vi "Unicode Path With LabVIEW File IO Example.vi"() -> ()   [LabVIEW 2020]
doc: "This example demonstrates creating and writing unicode paths using LabVIEW's TDMS primitives. This technique can be extended to any LabVIEW file I/O primitives such as config files, xml files, and so on."
uses:
  Unicode/Controls/String Encoding.ctl
  Types/UTF-8 String/UTF-8 String.lvclass/UTF-8 String.ctl
  Types/UTF-8 Path/UTF-8 Path.lvclass/UTF-8 Path.ctl
  adeaac51-e73f-479d-a693-bb7f399b7a58.vi
  c1cbc64f-dc2e-462b-b757-29338a356fe5.vi
  a3fedd63-8064-49e9-9d91-1abce6ab3d35.vi
  fc41487d-943f-4c2f-8ebb-b047207c64a4.vi
  Dialog & User Interface/Polymorphic VIs/Write Control Text/Write 1D String Array Value (UTF-8 String).vi
  3e39073b-8a5d-4733-9d90-f00b4091e0ed.vi
  Unicode/Encode String.vi
  adeaac51-e73f-479d-a693-bb7f399b7a58.vi/b0de225b-b813-4a3f-91fa-b2c78c384815.vi
  adeaac51-e73f-479d-a693-bb7f399b7a58.vi/b1dd94da-e188-4359-85d0-d6693b26af46.vi
  adeaac51-e73f-479d-a693-bb7f399b7a58.vi/2799960a-efad-449d-b375-cc5363f1c370.vi
  adeaac51-e73f-479d-a693-bb7f399b7a58.vi/2ed7adf8-1da0-426c-b32d-a1b4538e7e16.vi
  Types/UTF-8 String/Write Encoded UTF-8 String.vi
  Private/Conversion/Text as Encoded Path.vi
  Private/Conversion/Polymorphic VIs/Text as Encoded Path (UTF-8 String).vi
  Types/UTF-8 Path/Write Encoded UTF-8 Path.vi
  Private/Conversion/Path as Encoded Path.vi
  Private/Conversion/Polymorphic VIs/Path as Encoded Path (LabVIEW Path).vi
  Private/Conversion/Text as Encoded String.vi
  Private/Conversion/Polymorphic VIs/Text as Encoded String (UTF-8 Path).vi
  Private/Conversion/Path as UTF-8 Path.vi
  Private/Conversion/Polymorphic VIs/Path as UTF-8 Path (UTF-8 Path).vi
  Private/Library/gu_create_file.vi
  Private/Library/gu_long_path.vi
  Private/Conversion/Polymorphic VIs/Path as UTF-8 Path (LabVIEW Path).vi
  fc41487d-943f-4c2f-8ebb-b047207c64a4.vi/5269e09c-4216-478e-8686-9fb7d38e224a.vi
  fc41487d-943f-4c2f-8ebb-b047207c64a4.vi/d1f4a45d-6f02-44dd-a40b-2b28d80e6519.vi
  Private/Conversion/String as Encoded String.vi
  Private/Conversion/Polymorphic VIs/String as Encoded String (UTF-8 String).vi
  Private/Library/gu_list_folder.vi
  fc41487d-943f-4c2f-8ebb-b047207c64a4.vi/8eb4f0ed-0012-4550-978e-be3f7301df70.vi
  fc41487d-943f-4c2f-8ebb-b047207c64a4.vi/f7e6584c-01ed-423f-9bcd-660954191d0d.vi
  Private/Conversion/Polymorphic VIs/String as Encoded String (LabVIEW String).vi
  Dialog & User Interface/Polymorphic VIs/Write Control Text/Write 1D String Array Value (UTF-8 String).vi/5206cb6b-04fb-41f5-a37e-29c14f142303.vi
  3e39073b-8a5d-4733-9d90-f00b4091e0ed.vi/cd814f09-858d-41ec-a1ea-d598fdb95b0d.vi
  3e39073b-8a5d-4733-9d90-f00b4091e0ed.vi/cdde7a24-321d-4ebe-8fa8-ef041a4f6d83.vi
  Types/UTF-8 Path/New UTF-8 Path.vi
  Private/Library/gu_delete.vi
  3e39073b-8a5d-4733-9d90-f00b4091e0ed.vi/80924ba4-6f01-46cb-bebd-728ad922c70d.vi
  Private/Conversion/String as UTF-8 String.vi
  Private/Conversion/Polymorphic VIs/String as UTF-8 String (UTF-8 String).vi
  Private/Conversion/Text to UTF-8.vi
  Private/Conversion/Polymorphic VIs/Text to UTF-8 (LabVIEW String).vi
  Private/Conversion/Encoded UTF-8 String to Encoded UTF-16LE String.vi
  Private/Conversion/UTF-8 to Text.vi
  Private/Conversion/Polymorphic VIs/UTF-8 to Text (LabVIEW String).vi
  Private/Conversion/Encoded UTF-16LE String to Encoded UTF-8 String.vi
  Unicode/Prepend BOM.vi
  Types/UTF-8 String/Read Encoded UTF-8 String.vi
  Private/Conversion/Polymorphic VIs/Text to UTF-8 (LabVIEW Path).vi
  Types/UTF-8 Path/Read Encoded UTF-8 Path.vi
  Private/Library/Result To Error.vi
  Private/Memory/Copy String.vi
  fc41487d-943f-4c2f-8ebb-b047207c64a4.vi/5269e09c-4216-478e-8686-9fb7d38e224a.vi/c24c063b-f849-48a1-b323-238a063d7118.vi
  fc41487d-943f-4c2f-8ebb-b047207c64a4.vi/5269e09c-4216-478e-8686-9fb7d38e224a.vi/a2fd6c11-d594-45c9-8624-1f0a1df69df3.vi
  fc41487d-943f-4c2f-8ebb-b047207c64a4.vi/5269e09c-4216-478e-8686-9fb7d38e224a.vi/1fd3173e-d32e-42cb-8f0d-819132eb8e27.vi
  fc41487d-943f-4c2f-8ebb-b047207c64a4.vi/5269e09c-4216-478e-8686-9fb7d38e224a.vi/bb7c39fc-ad8e-447d-bc50-468674bfb562.vi
  fc41487d-943f-4c2f-8ebb-b047207c64a4.vi/8eb4f0ed-0012-4550-978e-be3f7301df70.vi/3a31b270-3bb6-4c58-a256-c5fcc2c98f09.vi
  fc41487d-943f-4c2f-8ebb-b047207c64a4.vi/8eb4f0ed-0012-4550-978e-be3f7301df70.vi/0ec5df2d-ef9b-4f84-a6a8-ffcedd45c4dc.vi
  Private/Conversion/Text as String.vi
  Private/Conversion/Polymorphic VIs/Text as String (UTF-8 Path).vi
  Private/Conversion/Polymorphic VIs/Text as Encoded String (UTF-8 String).vi
  3e39073b-8a5d-4733-9d90-f00b4091e0ed.vi/cd814f09-858d-41ec-a1ea-d598fdb95b0d.vi/9afeabe8-8abe-4536-bea1-05e5a3549c28.vi
  Private/Library/gu_open_file_dialog.vi
  Private/Library/gu_select_folder_dialog.vi
  Private/Conversion/Polymorphic VIs/Text as String (UTF-8 String).vi
  Unicode/SubVIs/Byte Order Marks.vi
  Unicode/Detect BOM.vi
  Private/Memory/Copy String.vi/4d47babd-4a2d-4eb7-b91b-7e707d692665.vi
  Private/Library/gu_free.vi
  Private/Conversion/Polymorphic VIs/Path as Encoded Path (UTF-8 Path).vi
  Private/Library/gu_string_subset.vi
  Private/Library/gu_to_lower_case.vi
  Private/Library/gu_search_split_string.vi
  Private/Conversion/Polymorphic VIs/Text as Encoded String (LabVIEW String).vi
  Unicode/Detect String Encoding.vi
  <vilib>/Utility/error.llb/Error Cluster From Error Code.vi
  Private/Memory/Copy String Array.vi
  Private/User Interface/Write String Array (1D).vi
  Types/UTF-8 String/UTF-8 String.lvclass
  Types/UTF-8 Path/UTF-8 Path.lvclass
  G-Unicode.lvlib
panel:
  out "error out":errorcluster
  out "TDMS Files":string[](array[string])
  # "Instructions:\n1. Run the VI.\n2. Check the TDMS Files contains a list of files with unicode characters."
  # "This example demonstrates creating and writing unicode paths using LabVIEW's TDMS primitives. This technique can be extended to any LabVIEW file I/O primitives such as config files, xml files, and so on.\n\nTo use unicode paths, it must first be converted to an 8.3 short path, which are compatible with any of LabVIEW's file I/O functions.\n\nIn order to convert the unicode path to the 8.3 short path, the file must first exist on disk. This can be achieved using Create File.vim, which accepts unicode paths.\n\nAfter file I/O is complete and the file closed, the short path can be converted back to the long (unicode) path."
  # "G"
  # "-Unicode"
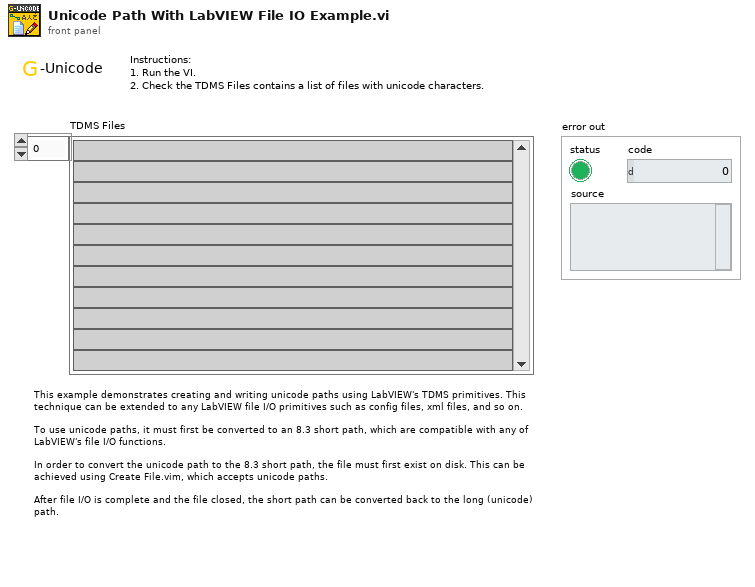
[diagram p1: front panel]
types:
  T1 = typedef "G-Unicode.lvlib/String Encoding.ctl" = enum16{"ANSI", "UTF-8", "UTF-16LE", "UTF-16BE", "Unknown"}
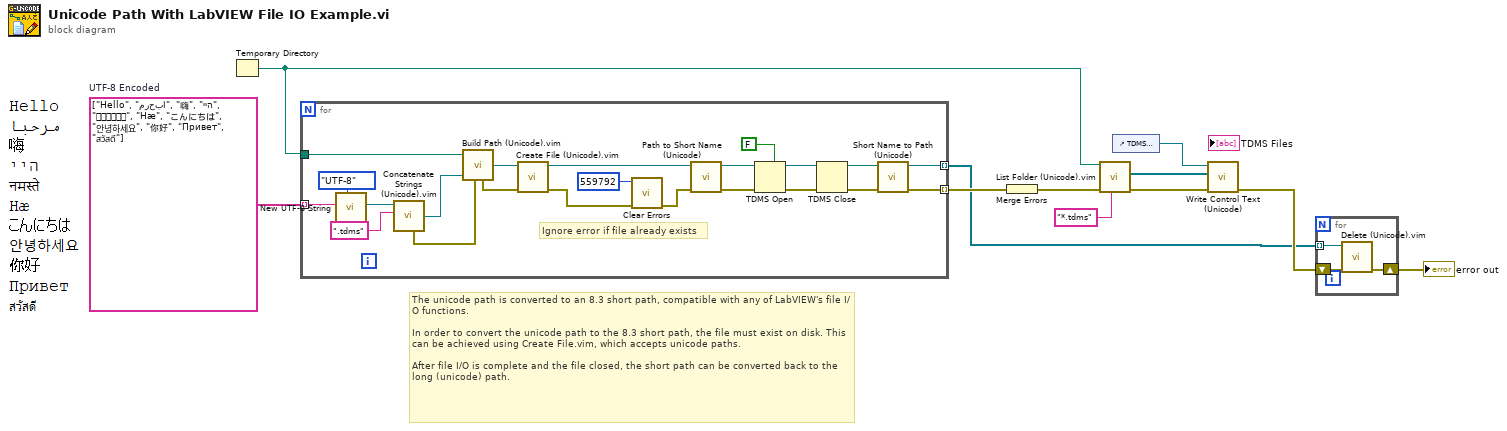
[diagram p0: block diagram]
diagram:
  w6 = string[] ["Hello", "مرحبا", "嗨", "היי", "नमस्ते", "Hæ", "こんにちは", "안녕하세요", "你好", "Привет", "สวัสดี"]  # UTF-8 Encoded
  # "The unicode path is converted to an 8.3 short path, compatible with any of LabVIEW's file I/O functions.\n\nIn order to convert the unicode path to the 8.3 short path, the file must exist on disk. This can be achieved using Create File.vim, which accepts unicode paths.\n\nAfter file I/O is complete and the file closed, the short path can be converted back to the long (unicode) path."
  n1 = Temporary Directory() -> (w3:path)
  n2 = for {
    tunnel: w3 -> [w24]
    tunnel: w6 -> [w19] mode=indexing
    tunnel: [w21] -> w8 mode=indexing
    tunnel: [w14] -> w4 mode=indexing
    # "Ignore error if file already exists"
    n3 = call "New UTF-8 String.vi"("Input Encoding (ANSI)"=String_Encoding."UTF-8", "String"=w19) -> ("UTF-8 String"=w18:refnum<class "UTF-8 String.lvclass">)  [unwired: 8 in, 1 out]
    n4 = call "Concatenate Strings (Unicode).vim"("Input 1"=".tdms" ("string"), "Input 0"=w18) -> ("error out"=w13:errorcluster, "Concatenated String"=w16:refnum<class "UTF-8 String.lvclass">)  [unwired: 7 in]
    n5 = call "Build Path (Unicode).vim"("Base Path"=w24, "Name or Relative Path"=w16, "error in"=w13) -> ("Appended Path"=w15:refnum<class "UTF-8 Path.lvclass">, "error out"=w22:errorcluster)  [unwired: 5 in]
    n6 = call "Create File (Unicode).vim"("error in"=w22, "Path"=w15) -> ("error out"=w33:errorcluster, "Path dup"=w31:refnum<class "UTF-8 Path.lvclass">)  [unwired: 8 in]
    n7 = call <vilib>:"Clear Errors.vi"("error in (no error)"=w33, "specific error code to clear (0: all)"=559792) -> ("error out"=w32:errorcluster)  [unwired: 4 in, 1 out]
    n8 = call "Path to Short Name (Unicode).vi"("error in"=w32, "Path"=w31) -> ("error out"=w29:errorcluster, "LabVIEW Path"=w30:path)  [unwired: 8 in]
    n9 = TDMS Open(5:FALSE ("create index file? (T)"), 8:w29, 11:w30) -> (0:w26:errorcluster, 3:w27:refnum<k34>)  [unwired: 4 in]
    n10 = TDMS Close(8:w26, 11:w27) -> (0:w23:errorcluster, 3:w25:path)
    n11 = call "Short Name to Path (Unicode).vi"("error in"=w23, "LabVIEW Path"=w25) -> ("error out"=w21:errorcluster, "UTF-8 Path"=w14:refnum<class "UTF-8 Path.lvclass">)  [unwired: 8 in]
  }
  n12 = Merge Errors(w8) -> (w7:errorcluster)
  n13 = call "List Folder (Unicode).vim"("Pattern"="*.tdms" ("string"), "error in"=w7, "Path"=w3) -> ("error out"=w9:errorcluster, "Filenames"=w10:refnum<class "UTF-8 String.lvclass">[])  [unwired: 5 in, 2 out]
  n14 = control-ref of="TDMS Files"() -> (w2:refnum<vi>)
  n15 = call-poly "Write Control Text (Unicode).vi"("error in"=w9, "Value"=w10, "Control Ref"=w2) -> ("error out"=w5:errorcluster)  [unwired: 8 in]
  n16 = for {
    shift-right: [w35] -> w1
    shift-left: w5 -> [w36]
    tunnel: w4 -> [w34] mode=indexing
    n17 = call "Delete (Unicode).vim"("error in"=w36, "Path"=w34) -> ("error out"=w35:errorcluster)  [unwired: 7 in, 2 out]
  }
  "error out" <- w1
